vi "DetectShutdownNotification.vi"(2 "error in (no error)":errorcluster, 3 "Shutdown Notifier":refnum<notifier>) -> (0 "error out":errorcluster, 1 "Shutdown":bool)   [LabVIEW 2013]
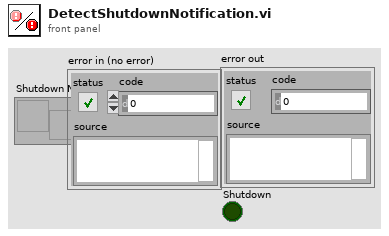
[diagram p1: front panel]
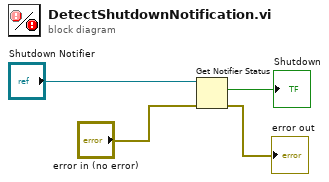
[diagram p0: block diagram]
diagram:
  n1 = Get Notifier Status(notifier="Shutdown Notifier", error in (no error)="error in (no error)") -> (current notification=→"Shutdown":bool, error out=→"error out":errorcluster)  [unwired: 3 out]
